vi "rszvl_core_global.vi"() -> ()   [LabVIEW 2014] (continued)
measured frequencies or whether an ENR list table is to be used (ENR values specified at specific input frequencies).\n\nAvailable Repeated Capabilities:\nNone\n\nRemote-control command(s):\n[SENSe]:CORRection:ENR:MODE[?] TABLe | SPOT", "Flags"={"OPC Wait"=FALSE, "Dont check status"=FALSE, "*WAI"=FALSE}, "Check Status Callback"=""}, {"Level"=3, "Descriptive Name"="Noise ERN Constant Value", "Class Only"=FALSE, "Data Type"=1, "Access"=2, "Identifier"="RSZVL_ATTR_NOISE_CORR_ENR_SPOT", "Range Table"="", "Command"="SENS:CORR:ENR:SPOT", "Read Callback"="", "Write Callback"="", "Range Callback"="", "Check Callback"="", "Rngtable Callback"="", "Coerce Callback"="", "User Callback"="", "Supported Models"="", "Instrument Options"="", "Repeated Capabilities"="", "Restricted Repeated Capabilities"="", "Help"="The ENR attribute allows the ENR value applicable to the Noise source for all input frequencies to be specified. This value provides a simple mechanism to enter an ENR value that is\napplicable throughout a range of measurement frequencies.\nThis attribute will however not be effective if\nthe remote control command SENS:CORR:ENR:MODE:TABL was previously entered.\n\nAvailable Repeated Capabilities:\nNone\n\nRemote-control command(s):\n[SENSe]:CORRection:ENR:SPOT[?] <numeric_value> [dB]", "Flags"={"OPC Wait"=FALSE, "Dont check status"=FALSE, "*WAI"=FALSE}, "Check Status Callback"=""}, {"Level"=3, "Descriptive Name"="Noise ENR Room Temperature", "Class Only"=FALSE, "Data Type"=1, "Access"=2, "Identifier"="RSZVL_ATTR_NOISE_CORR_TEMP", "Range Table"="", "Command"="SENS:CORR:TEMP", "Read Callback"="", "Write Callback"="", "Range Callback"="", "Check Callback"="", "Rngtable Callback"="", "Coerce Callback"="", "User Callback"="", "Supported Models"="", "Instrument Options"="", "Repeated Capabilities"="", "Restricted Repeated Capabilities"="", "Help"="This ENR attribute allows the room temperature of the operating environment to be specified. This value will be taken into account when calculating noise results. Units are Kelvin.\n\nAvailable Repeated Capabilities:\nNone\n\nRemote-control command(s):\n[SENSe]:CORRection:TEMPerature[?] <numeric_value> [K]", "Flags"={"OPC Wait"=FALSE, "Dont check status"=FALSE, "*WAI"=FALSE}, "Check Status Callback"=""}, {"Level"=3, "Descriptive Name"="Noise Loss Mode Selection", "Class Only"=FALSE, "Data Type"=0, "Access"=2, "Identifier"="RSZVL_ATTR_NOISE_CORR_LOSS_MODE", "Range Table"="rszvl_rngNoiseLossMode", "Command"="SENS:CORR:LOSS:{InputOutput}:MODE", "Read Callback"="", "Write Callback"="", "Range Callback"="", "Check Callback"="", "Rngtable Callback"="", "Coerce Callback"="", "User Callback"="", "Supported Models"="", "Instrument Options"="", "Repeated Capabilities"="", "Restricted Repeated Capabilities"="", "Help"="This attribute is used to identify whether a single input/output loss value applies for all measured frequencies or whether an input/output loss list is to be used. (Loss Input/Output values specified at specific input frequencies).\n\nAvailable Repeated Capabilities:\nInputOutput: Inp,Out\r\n\nRemote-control command(s):\n[SENSe]:CORRection:LOSS:INPut|OUTput:MODE[?] SPOT | TABLe", "Flags"={"OPC Wait"=FALSE, "Dont check status"=FALSE, "*WAI"=FALSE}, "Check Status Callback"=""}, {"Level"=3, "Descriptive Name"="Noise Loss Constant Value", "Class Only"=FALSE, "Data Type"=1, "Access"=2, "Identifier"="RSZVL_ATTR_NOISE_CORR_LOSS_SPOT", "Range Table"="", "Command"="SENS:CORR:LOSS:{InputOutput}:SPOT", "Read Callback"="", "Write Callback"="", "Range Callback"="", "Check Callback"="", "Rngtable Callback"="", "Coerce Callback"="", "User Callback"="", "Supported Models"="", "Instrument Options"="", "Repeated Capabilities"="", "Restricted Repeated Capabilities"="", "Help"="This attribute allows the loss input/output constant to be set to a value applicable for all input/output frequencies to be measured. This attribute provides a simple mechanism to enter a loss input/output value that is applicable throughout a range of measurement frequencies.\nThis attribute will however not be effective if the attribute RSZVL_ATTR_NOISE_CORR_LOSS_MODE - TABL was previously entered.\n\nAvailable Repeated Capabilities:\nInputOutput: Inp,Out\r\n\nRemote-control command(s):\n[SENSe]:CORRection:LOSS:<INPut|OUTPut>:SPOT[?] <numeric value> [dB]", "Flags"={"OPC Wait"=FALSE, "Dont check status"=FALSE, "*WAI"=FALSE}, "Check Status Callback"=""}, {"Level"=3, "Descriptive Name"="Noise Image Rejection", "Class Only"=FALSE, "Data Type"=1, "Access"=2, "Identifier"="RSZVL_ATTR_NOISE_CORR_EREJ", "Range Table"="", "Command"="SENS:CORR:IREJ", "Read Callback"="", "Write Callback"="", "Range Callback"="", "Check Callback"="", "Rngtable Callback"="", "Coerce Callback"="", "User Callback"="", "Supported Models"="", "Instrument Options"="", "Repeated Capabilities"="", "Restricted Repeated Capabilities"="", "Help"="This attribute allows an image rejection value associated with DUT to be entered which will be effective across the complete range of measurement frequencies.\n\nAvailable Repeated Capabilities:\nNone\n\nRemote-control command(s):\n[SENSe]:CORRection:IREJection[?] <numeric value > [dB]", "Flags"={"OPC Wait"=FALSE, "Dont check status"=FALSE, "*WAI"=FALSE}, "Check Status Callback"=""}, {"Level"=3, "Descriptive Name"="Noise 2nd State Correction", "Class Only"=FALSE, "Data Type"=3, "Access"=2, "Identifier"="RSZVL_ATTR_NOISE_CORR_STAT", "Range Table"="", "Command"="SENS:CORR:STAT", "Read Callback"="", "Write Callback"="", "Range Callback"="", "Check Callback"="", "Rngtable Callback"="", "Coerce Callback"="", "User Callback"="", "Supported Models"="", "Instrument Options"="", "Repeated Capabilities"="", "Restricted Repeated Capabilities"="", "Help"="This attribute can be used to control whether the R&S FS-K30 option will factor in the results obtained from second stage correction when performing a noise and gain measurement.\n\nAvailable Repeated Capabilities:\nNone\n\nRemote-control command(s):\n[SENSe]:CORRection[:STATe][?] ON | OFF", "Flags"={"OPC Wait"=FALSE, "Dont check status"=FALSE, "*WAI"=FALSE}, "Check Status Callback"=""}, {"Level"=3, "Descriptive Name"="Noise Frequency Step", "Class Only"=FALSE, "Data Type"=1, "Access"=2, "Identifier"="RSZVL_ATTR_NOISE_FREQ_STEP", "Range Table"="", "Command"="SENS:FREQ:STEP", "Read Callback"="", "Write Callback"="", "Range Callback"="", "Check Callback"="", "Rngtable Callback"="", "Coerce Callback"="", "User Callback"="", "Supported Models"="", "Instrument Options"="", "Repeated Capabilities"="", "Restricted Repeated Capabilities"="", "Help"="This attribute can be used to specify the step frequency for a new frequency measurement list that requires computing. This value will form the basis of one of the input criteria for computing a new frequency list.\n\nAvailable Repeated Capabilities:\nNone\n\nRemote-control command(s):\n[SENSe]:FREQuency:STEP[?] <numeric value> [Hz]", "Flags"={"OPC Wait"=FALSE, "Dont check status"=FALSE, "*WAI"=FALSE}, "Check Status Callback"=""}, {"Level"=3, "Descriptive Name"="Noise Fixed Frequency", "Class Only"=FALSE, "Data Type"=1, "Access"=2, "Identifier"="RSZVL_ATTR_NOISE_FREQ_FIXED", "Range Table"="", "Command"="SENS:FREQ:FIX", "Read Callback"="", "Write Callback"="", "Range Callback"="", "Check Callback"="", "Rngtable Callback"="", "Coerce Callback"="", "User Callback"="", "Supported Models"="", "Instrument Options"="", "Repeated Capabilities"="", "Restricted Repeated Capabilities"="", "Help"="This attribute is used to specify a single fixed frequency to measure noise and gain continuously. The value specified with this command is only used when a single frequency measurement is initiated.\n\nAvailable Repeated Capabilities:\nNone\n\nRemote-control command(s):\n[SENSe]:FREQuency[:CW|:FIXed][?] <numeric value> [Hz]", "Flags"={"OPC Wait"=FALSE, "Dont check status"=FALSE, "*WAI"=FALSE}, "Check Status Callback"=""}, {"Level"=3, "Descriptive Name"="Noise Fixed Local Oscilator Frequency", "Class Only"=FALSE, "Data Type"=1, "Access"=2, "Identifier"="RSZVL_ATTR_NOISE_CONF_SYST_LOSC_FREQ", "Range Table"="", "Command"="SENS:CONF:MODE:SYST:LOSC:FREQ", "Read Callback"="", "Write Callback"="", "Range Callback"="", "Check Callback"="", "Rngtable Callback"="", "Coerce Callback"="", "User Callback"="", "Supported Models"="", "Instrument Options"="", "Repeated Capabilities"="", "Restricted Repeated Capabilities"="", "Help"="This attribute can be used to specify a fixed local oscillator frequency for a new frequency measurement list that requires computing. This value will form the basis of one of the input criteria for computing a new frequency list.\nThe attribute will not have any immediate effect if a direct frequency list is being used (which is set by the RSZVL_ATTR_NOISE_CONF_MODE_DUT - AMPL attribute) or a variable local osciallator frequency has been specified (which is set by the RSZVL_ATTR_NOISE_CONF_SYST_LOSC - VAR attribute).\n\nAvailable Repeated Capabilities:\nNone\n\nRemote-control command(s):\n[SENSe]:CONFigure:MODE:SYSTem:LOSCillator:FREQuency[?] <numeric value> [Hz]", "Flags"={"OPC Wait"=FALSE, "Dont check status"=FALSE, "*WAI"=FALSE}, "Check Status Callback"=""}, {"Level"=3, "Descriptive Name"="Noise Configure DUT", "Class Only"=FALSE, "Data Type"=0, "Access"=2, "Identifier"="RSZVL_ATTR_NOISE_CONF_MODE_DUT", "Range Table"="rszvl_rngNoiseConfDUT", "Command"="SENS:CONF:MODE:DUT", "Read Callback"="", "Write Callback"="", "Range Callback"="", "Check Callback"="", "Rngtable Callback"="", "Coerce Callback"="", "User Callback"="", "Supported Models"="", "Instrument Options"="", "Repeated Capabilities"="", "Restricted Repeated Capabilities"="", "Help"="This attribute allows the type of DUT to be defined. This setting will determine the method that will be used to create the frequency measurement list. This attribute in addition to Noise Configure Local Oscilator will determine how the DUT is tested. Fixed Local Oscillator or fixed Intermediate Frequencies will be taken from the settings supplied by its functions, where appropriate.\nThe following calculation methods will be used.\nUsing a variable Local Oscillator frequency as set by the attribute RSZVL_ATTR_NOISE_CONF_SYST_LOSC - VAR: i.e. the DUT has a fixed IF frequency.\nUsing a fixed Local Oscillator frequency as set by the attribute RSZVL_ATTR_NOISE_CONF_SYST_LOSC -\nFIX: i.e. the DUT has a variable IF frequency.\nThe attribute will not have any immediate effect if the current frequency measurement mode is\nfixed, as is set by the command SENS:FREQ:MODE FIX.\nRF: = All the above settings for frequency list calculation will calculate the RF frequency for each step.\nThe list of RF frequencies generated will be in the following sequence: Start Frequency, Start\nFrequency + Step Frequency, Start Frequency + Step Frequency*2, Stop Frequency.\nIF: = intermediate frequency\nLO: = local oscillator frequency\n\nAvailable Repeated Capabilities:\nNone\n\nRemote-control command(s):\n[SENSe]:CONFigure:MODE:DUT[?] AMPLifier | DOWNc | UPConv", "Flags"={"OPC Wait"=FALSE, "Dont check status"=FALSE, "*WAI"=FALSE}, "Check Status Callback"=""}, {"Level"=3, "Descriptive Name"="Noise Configure Range", "Class Only"=FALSE, "Data Type"=1, "Access"=2, "Identifier"="RSZVL_ATTR_NOISE_CONF_DUT_GAIN", "Range Table"="", "Command"="SYST:CONF:DUT:GAIN", "Read Callback"="", "Write Callback"="", "Range Callback"="", "Check Callback"="", "Rngtable Callback"="", "Coerce Callback"="", "User Callback"="", "Supported Models"="", "Instrument Options"="", "Repeated Capabilities"="", "Restricted Repeated Capabilities"="", "Help"="This attribute allows the maximum gain of the DUT to be specified.\n\nAvailable Repeated Capabilities:\nNone\n\nRemote-control command(s):\nSYSTem:CONFigure:DUT:GAIN[?] <numeric value> [dB]", "Flags"={"OPC Wait"=FALSE, "Dont check status"=FALSE, "*WAI"=FALSE}, "Check Status Callback"=""}, {"Level"=3, "Descriptive Name"="Noise Settling Time", "Class Only"=FALSE, "Data Type"=1, "Access"=2, "Identifier"="RSZVL_ATTR_NOISE_CONF_DUT_SETT_TIME", "Range Table"="", "Command"="SYST:CONF:DUT:STIM", "Read Callback"="", "Write Callback"="", "Range Callback"="", "Check Callback"="", "Rngtable Callback"="", "Coerce Callback"="", "User Callback"="", "Supported Models"="", "Instrument Options"="", "Repeated Capabilities"="", "Restricted Repeated Capabilities"="", "Help"="This attribute allows the DUT settling time to be modified. It represents the time to wait for the DUT to settle after a noise source has been turned on or off.\n\nAvailable Repeated Capabilities:\nNone\n\nRemote-control command(s):\nSYSTem:CONFigure:DUT:STIMe[?] <numeric value> [s]", "Flags"={"OPC Wait"=FALSE, "Dont check status"=FALSE, "*WAI"=FALSE}, "Check Status Callback"=""}, {"Level"=3, "Descriptive Name"="Noise Save Trace To Memory", "Class Only"=FALSE, "Data Type"=4, "Access"=1, "Identifier"="RSZVL_ATTR_NOISE_ARRAY_MEMORY", "Range Table"="", "Command"="CONF:ARR:MEM{NoiseTraceMemory} ONCE", "Read Callback"="", "Write Callback"="", "Range Callback"="", "Check Callback"="", "Rngtable Callback"="", "Coerce Callback"="", "User Callback"="", "Supported Models"="", "Instrument Options"="", "Repeated Capabilities"="", "Restricted Repeated Capabilities"="", "Help"="This attribute saves the current trace results (noise figure, noise temperature and noise gain traces) to trace memory <n>.\n\nAvailable Repeated Capabilities:\nNoiseTraceMemory: MEM1,MEM2,MEM3\r\n\nRemote-control command(s):\nCONFigure:ARRay:MEMory<1...3> ONCE", "Flags"={"OPC Wait"=FALSE, "Dont check status"=FALSE, "*WAI"=FALSE}, "Check Status Callback"=""}, {"Level"=3, "Descriptive Name"="Noise Assign Marker To Trace", "Class Only"=FALSE, "Data Type"=0, "Access"=2, "Identifier"="RSZVL_ATTR_NOISE_MARKER_TRACE", "Range Table"="rszvl_rngNoiseMarkerTrace", "Command"="CALC:MARK:TRAC", "Read Callback"="", "Write Callback"="", "Range Callback"="", "Check Callback"="", "Rngtable Callback"="", "Coerce Callback"="", "User Callback"="", "Supported Models"="", "Instrument Options"="", "Repeated Capabilities"="", "Restricted Repeated Capabilities"="", "Help"="This attribute assigns the marker1 to the indicated trace.\n\nAvailable Repeated Capabilities:\nNone\n\nRemote-control command(s):\nCALCulate:MARKer:TRACe NOISe | GAIN", "Flags"={"OPC Wait"=FALSE, "Dont check status"=FALSE, "*WAI"=FALSE}, "Check Status Callback"=""}, {"Level"=2, "Descriptive Name"="Display", "Class Only"=TRUE, "Data Type"=0, "Access"=0, "Identifier"="", "Range Table"="", "Command"="", "Read Callback"="", "Write Callback"="", "Range Callback"="", "Check Callback"="", "Rngtable Callback"="", "Coerce Callback"="", "User Callback"="", "Supported Models"="", "Instrument Options"="", "Repeated Capabilities"="", "Restricted Repeated Capabilities"="", "Help"="Attributes that configure the display parameters.\n\n(1) Noise Display Y-Axis Trace Type:\nThis attribute allows the user to specify the type of data to be displayed in trace 1. The user can select either to display either Noise Figure results (NFIGure) or Noise temperature (TEFFective – to keep compatibility with the NFA). Note that Trace 1 is always noise results and Trace 2 is always for Gain results.\n\n(2) Noise Display Trace State:\nThis attribute switches on or off the display of the corresponding trace and related information in\nthe selected measurement window.\n\n(3) Noise Display Symbols:\nThis attribute switches on or off the display of the symbols to mark the measurement points for the\nspecified trace i.e. Noise or Gain.\nThis attribute will only have a noticeable effect if the required trace is active as set by the\nattribute RSZVL_ATTR_NOISE_DISP_TRAC_STAT ON.\n\n(4) Noise Automatic Scaling:\nThis attribute switches on or off automatic scaling of the Y-axis for the specified trace display.\nAutomatic scaling set the Y-axis to automatically scale to best fit the measurement results.\nNote that the specified trace must be active for this attribute to have an immediate effect. This can be achieved using the attribute RSZVL_ATTR_NOISE_DISP_TRAC_STAT ON.\n\n(5) Noise Minimum Y-Axis Value:\nThis attribute sets the minimum (bottom) Y-axis display value for the specified trace display. Note that this attribute has no affect if automatic scaling of the Y-axis is enabled or the specified trace is not currently active.\n\n(6) Noise Maximum Y-Axis Value:\nThis attribute sets the maximum (top) Y-axis display value for the specified trace display. Note that this attribute has no affect if automatic scaling of the Y-axis is enabled or the specified trace is not currently active.\n\n(7) Noise Automatic Reference Level:\nThis attribute enables or disables automatic reference level detection.\n\n(8) Noise Display Table:\nThis attribute toggles the display of results in graphical or tabular form.\n\n(9) Noise Display Trace Memory:\nswitches the display of trace memory <n> on or off.\nThis command is available from firmware version 1.60.\n\n(10) Noise Display Current Results State:\nThis attribute switches the display of the current measurement results on or off.\nThis command is available from firmware version 1.60.\n\n(11) Noise X-Axis Frequency Display:\nThis attribute selects the frequency to be displayed on the x–axis if the DUT is not an amplifier, i.e. in a frequency–converting measurement mode.", "Flags"={"OPC Wait"=FALSE, "Dont check status"=FALSE, "*WAI"=FALSE}, "Check Status Callback"=""}, {"Level"=3, "Descriptive Name"="Noise Display Y-Axis Trace Type", "Class Only"=FALSE, "Data Type"=0, "Access"=2, "Identifier"="RSZVL_ATTR_NOISE_DISP_DATA_TRAC", "Range Table"="rszvl_rngNoiseDispDataTrac", "Command"="DISP:DATA:TRAC{Trace}", "Read Callback"="", "Write Callback"="", "Range Callback"="", "Check Callback"="", "Rngtable Callback"="", "Coerce Callback"="", "User Callback"="", "Supported Models"="", "Instrument Options"="", "Repeated Capabilities"="", "Restricted Repeated Capabilities"="", "Help"="This attribute allows the user to specify the type of data to be displayed in trace 1. The user can select either to display either Noise Figure results (NFIGure) or Noise temperature (TEFFective – to keep compatibility with the NFA). Note that Trace 1 is always noise results and Trace 2 is always for Gain results.\n\nAvailable Repeated Capabilities:\nTrace: TR1,TR2,TR3,TR4,TR5,TR6,TR7,TR8,TR9,TR10,TR11,TR12,TR13,TR14,TR15,TR16,TR17,TR18,TR19,TR20\r\n\nRemote-control command(s):\nDISPlay:DATA:TRACe<1>[?] NFIGure | TEFFective", "Flags"={"OPC Wait"=FALSE, "Dont check status"=FALSE, "*WAI"=FALSE}, "Check Status Callback"=""}, {"Level"=3, "Descriptive Name"="Noise Display Trace State", "Class Only"=FALSE, "Data Type"=3, "Access"=2, "Identifier"="RSZVL_ATTR_NOISE_DISP_TRAC_STAT", "Range Table"="", "Command"="DISP:TRAC{Trace}", "Read Callback"="", "Write Callback"="", "Range Callback"="", "Check Callback"="", "Rngtable Callback"="", "Coerce Callback"="", "User Callback"="", "Supported Models"="", "Instrument Options"="", "Repeated Capabilities"="", "Restricted Repeated Capabilities"="", "Help"="This attribute switches on or off the display of the corresponding trace and related information in\nthe selected measurement window.\n\nAvailable Repeated Capabilities:\nTrace: TR1,TR2,TR3,TR4,TR5,TR6,TR7,TR8,TR9,TR10,TR11,TR12,TR13,TR14,TR15,TR16,TR17,TR18,TR19,TR20\r\n\nRemote-control command(s):\nDISPlay[:WINDow<1>]:TRACe<1|2>[:STATe][?] ON | OFF", "Flags"={"OPC Wait"=FALSE, "Dont check status"=FALSE, "*WAI"=FALSE}, "Check Status Callback"=""}, {"Level"=3, "Descriptive Name"="Noise Display Symbols", "Class Only"=FALSE, "Data Type"=3, "Access"=2, "Identifier"="RSZVL_ATTR_NOISE_DISP_SYMB", "Range Table"="", "Command"="DISP:TRAC{Trace}:SYMB", "Read Callback"="", "Write Callback"="", "Range Callback"="", "Check Callback"="", "Rngtable Callback"="", "Coerce Callback"="", "User Callback"="", "Supported Models"="", "Instrument Options"="", "Repeated Capabilities"="", "Restricted Repeated Capabilities"="", "Help"="This attribute switches on or off the display of the symbols to mark the measurement points for the\nspecified trace i.e. Noise or Gain.\nThis attribute will only have a noticeable effect if the required trace is active as set by the\nattribute RSZVL_ATTR_NOISE_DISP_TRAC_STAT ON.\n\nAvailable Repeated Capabilities:\nTrace: TR1,TR2,TR3,TR4,TR5,TR6,TR7,TR8,TR9,TR10,TR11,TR12,TR13,TR14,TR15,TR16,TR17,TR18,TR19,TR20\r\n\nRemote-control command(s):\nDISPlay[:WINDow<1>]:TRACe<1|2>:SYMBols[?] ON | OFF", "Flags"={"OPC Wait"=FALSE, "Dont check status"=FALSE, "*WAI"=FALSE}, "Check Status Callback"=""}, {"Level"=3, "Descriptive Name"="Noise Automatic Scaling", "Class Only"=FALSE, "Data Type"=3, "Access"=2, "Identifier"="RSZVL_ATTR_NOISE_DISP_AUTO_SCAL", "Range Table"="", "Command"="DISP:TRAC{Trace}:Y:AUTO", "Read Callback"="", "Write Callback"="", "Range Callback"="", "Check Callback"="", "Rngtable Callback"="", "Coerce Callback"="", "User Callback"="", "Supported Models"="", "Instrument Options"="", "Repeated Capabilities"="", "Restricted Repeated Capabilities"="", "Help"="This attribute switches on or off automatic scaling of the Y-axis for the specified trace display.\nAutomatic scaling set the Y-axis to automatically scale to best fit the measurement results.\nNote that the specified trace must be active for this attribute to have an immediate effect. This can be achieved using the attribute RSZVL_ATTR_NOISE_DISP_TRAC_STAT ON.\n\nAvailable Repeated Capabilities:\nTrace: TR1,TR2,TR3,TR4,TR5,TR6,TR7,TR8,TR9,TR10,TR11,TR12,TR13,TR14,TR15,TR16,TR17,TR18,TR19,TR20\r\n\nRemote-control command(s):\nDISPlay[:WINDow<1>]:TRACe<1|2>:Y[:SCALe]:AUTO[?] ON | OFF", "Flags"={"OPC Wait"=FALSE, "Dont check status"=FALSE, "*WAI"=FALSE}, "Check Status Callback"=""}, {"Level"=3, "Descriptive Name"="Noise Minimum Y-Axis Value", "Class Only"=FALSE, "Data Type"=1, "Access"=2, "Identifier"="RSZVL_ATTR_NOISE_DISP_TRAC_BOTTOM", "Range Table"="", "Command"="DISP:TRAC{Trace}:Y:BOTT", "Read Callback"="", "Write Callback"="", "Range Callback"="", "Check Callback"="", "Rngtable Callback"="", "Coerce Callback"="", "User Callback"="", "Supported Models"="", "Instrument Options"="", "Repeated Capabilities"="", "Restricted Repeated Capabilities"="", "Help"="This attribute sets the minimum (bottom) Y-axis display value for the specified trace display. Note that this attribute has no affect if automatic scaling of the Y-axis is enabled or the specified trace is not currently active.\n\nAvailable Repeated Capabilities:\nTrace: TR1,TR2,TR3,TR4,TR5,TR6,TR7,TR8,TR9,TR10,TR11,TR12,TR13,TR14,TR15,TR16,TR17,TR18,TR19,TR20\r\n\nRemote-control command(s):\nDISPlay[:WINDow<1>]:TRACe<1|2>:Y[:SCALe]:BOTTom[?] <numeric_value> [dB]", "Flags"={"OPC Wait"=FALSE, "Dont check status"=FALSE, "*WAI"=FALSE}, "Check Status Callback"=""}, {"Level"=3, "Descriptive Name"="Noise Maximum Y-Axis Value", "Class Only"=FALSE, "Data Type"=1, "Access"=2, "Identifier"="RSZVL_ATTR_NOISE_DISP_TRAC_TOP", "Range Table"="", "Command"="DISP:TRAC{Trace}:Y:TOP", "Read Callback"="", "Write Callback"="", "Range Callback"="", "Check Callback"="", "Rngtable Callback"="", "Coerce Callback"="", "User Callback"="", "Supported Models"="", "Instrument Options"="", "Repeated Capabilities"="", "Restricted Repeated Capabilities"="", "Help"="This attribute sets the maximum (top) Y-axis display value for the specified trace display. Note that this attribute has no affect if automatic scaling of the Y-axis is enabled or the specified trace is not currently active.\n\nAvailable Repeated Capabilities:\nTrace: TR1,TR2,TR3,TR4,TR5,TR6,TR7,TR8,TR9,TR10,TR11,TR12,TR13,TR14,TR15,TR16,TR17,TR18,TR19,TR20\r\n\nRemote-control command(s):\nDISPlay[:WINDow<1>]:TRACe<1|2>:Y[:SCALe]:TOP[?] <numeric_value> [dB]", "Flags"={"OPC Wait"=FALSE, "Dont check status"=FALSE, "*WAI"=FALSE}, "Check Status Callback"=""}, {"Level"=3, "Descriptive Name"="Noise Automatic Reference Level", "Class Only"=FALSE, "Data Type"=3, "Access"=2, "Identifier"="RSZVL_ATTR_NOISE_DISP_TRAC_REF_LEV_STAT", "Range Table"="", "Command"="DISP:TRAC{Trace}:Y:RLEV:AUTO", "Read Callback"="", "Write Callback"="", "Range Callback"="", "Check Callback"="", "Rngtable Callback"="", "Coerce Callback"="", "User Callback"="", "Supported Models"="", "Instrument Options"="", "Repeated Capabilities"="", "Restricted Repeated Capabilities"="", "Help"="This attribute enables or disables automatic reference level detection.\n\nAvailable Repeated Capabilities:\nTrace: TR1,TR2,TR3,TR4,TR5,TR6,TR7,TR8,TR9,TR10,TR11,TR12,TR13,TR14,TR15,TR16,TR17,TR18,TR19,TR20\r\n\nRemote-control command(s):\nDISPlay[:WINDow<1>]:TRACe<1|2>:Y[:SCALe]:RLEVel:AUTO[?] ON | OFF", "Flags"={"OPC Wait"=TRUE, "Dont check status"=FALSE, "*WAI"=FALSE}, "Check Status Callback"=""}, {"Level"=3, "Descriptive Name"="Display Format", "Class Only"=FALSE, "Data Type"=0, "Access"=2, "Identifier"="RSZVL_ATTR_NOISE_DISP_FORMAT", "Range Table"="rszvl_rngDISPFormat", "Command"="DISP:FORM", "Read Callback"="", "Write Callback"="", "Range Callback"="", "Check Callback"="", "Rngtable Callback"="", "Coerce Callback"="", "User Callback"="", "Supported Models"="", "Instrument Options"="", "Repeated Capabilities"="", "Restricted Repeated Capabilities"="", "Help"="This attribute switches the measurement result display between FULL SCREEN and SPLIT SCREEN. The coupling of settings between screen A and screen B can be selected with the command INSTrument:COUPle.\n\nAvailable Repeated Capabilities:\nNone\n\nRemote-control command(s):\nDISPlay:FORMat SINGle | SPLit", "Flags"={"OPC Wait"=FALSE, "Dont check status"=FALSE, "*WAI"=FALSE}, "Check Status Callback"=""}, {"Level"=3, "Descriptive Name"="Noise Display Table", "Class Only"=FALSE, "Data Type"=3, "Access"=2, "Identifier"="RSZVL_ATTR_NOISE_DISP_TABLE", "Range Table"="", "Command"="DISP:TABL", "Read Callback"="", "Write Callback"="", "Range Callback"="", "Check Callback"="", "Rngtable Callback"="", "Coerce Callback"="", "User Callback"="", "Supported Models"="", "Instrument Options"="", "Repeated Capabilities"="", "Restricted Repeated Capabilities"="", "Help"="This attribute toggles the display of results in graphical or tabular form.\n\nAvailable Repeated Capabilities:\nNone\n\nRemote-control command(s):\nDISPlay[:WINDow<1>]:TABLe[?] ON | OFF", "Flags"={"OPC Wait"=FALSE, "Dont check status"=FALSE, "*WAI"=FALSE}, "Check Status Callback"=""}, {"Level"=3, "Descriptive Name"="Noise Display Trace Memory", "Class Only"=FALSE, "Data Type"=3, "Access"=2, "Identifier"="RSZVL_ATTR_NOISE_DISP_TRACE_MEM", "Range Table"="", "Command"="DISP:ARR:MEM{NoiseTraceMemory}", "Read Callback"="", "Write Callback"="", "Range Callback"="", "Check Callback"="", "Rngtable Callback"="", "Coerce Callback"="", "User Callback"="", "Supported Models"="", "Instrument Options"="", "Repeated Capabilities"="", "Restricted Repeated Capabilities"="", "Help"="switches the display of trace memory <n> on or off.\nThis command is available from firmware version 1.60.\n\nAvailable Repeated Capabilities:\nNoiseTraceMemory: MEM1,MEM2,MEM3\r\n\nRemote-control command(s):\nDISPlay:ARRay:MEMory<1...3>[:STATe]", "Flags"={"OPC Wait"=FALSE, "Dont check status"=FALSE, "*WAI"=FALSE}, "Check Status Callback"=""}, {"Level"=3, "Descriptive Name"="Noise Display Current Results State", "Class Only"=FALSE, "Data Type"=3, "Access"=2, "Identifier"="RSZVL_ATTR_NOISE_DISPL_CURR_RESULTS", "Range Table"="", "Command"="DISP:CURR:DATA", "Read Callback"="", "Write Callback"="", "Range Callback"="", "Check Callback"="", "Rngtable Callback"="", "Coerce Callback"="", "User Callback"="", "Supported Models"="", "Instrument Options"="", "Repeated Capabilities"="", "Restricted Repeated Capabilities"="", "Help"="This attribute switches the display of the current measurement results on or off.\nThis command is available from firmware version 1.60.\n\nAvailable Repeated Capabilities:\nNone\n\nRemote-control command(s):\nDISPlay:CURRent:DATA[:STATe] OFF | ON", "Flags"={"OPC Wait"=FALSE, "Dont check status"=FALSE, "*WAI"=FALSE}, "Check Status Callback"=""}, {"Level"=3, "Descriptive Name"="Noise X-Axis Frequency Display", "Class Only"=FALSE, "Data Type"=0, "Access"=2, "Identifier"="RSZVL_ATTR_NOISE_DISP_X_AXIS", "Range Table"="rszvl_rngNoiseXAxisFrequency", "Command"="DISP:TRAC{Trace}:X", "Read Callback"="", "Write Callback"="", "Range Callback"="", "Check Callback"="", "Rngtable Callback"="", "Coerce Callback"="", "User Callback"="", "Supported Models"="", "Instrument Options"="", "Repeated Capabilities"="", "Restricted Repeated Capabilities"="", "Help"="This attribute selects the frequency to be displayed on the x–axis if the DUT is not an amplifier, i.e. in a frequency–converting measurement mode.\n\nAvailable Repeated Capabilities:\nTrace: TR1,TR2,TR3,TR4,TR5,TR6,TR7,TR8,TR9,TR10,TR11,TR12,TR13,TR14,TR15,TR16,TR17,TR18,TR19,TR20\r\n\nRemote-control command(s):\nDISPlay[:WINDow<1>]:TRACe<1|2>:X[:SCALe]", "Flags"={"OPC Wait"=FALSE, "Dont check status"=FALSE, "*WAI"=FALSE}, "Check Status Callback"=""}, {"Level"=1, "Descriptive Name"="K72 - 3GPP FDD Base Station Test", "Class Only"=TRUE, "Data Type"=0, "Access"=0, "Identifier"="", "Range Table"="", "Command"="", "Read Callback"="", "Write Callback"="", "Range Callback"="", "Check Callback"="", "Rngtable Callback"="", "Coerce Callback"="", "User Callback"="", "Supported Models"="", "Instrument Options"="", "Repeated Capabilities"="", "Restricted Repeated Capabilities"="", "Help"="This class implements attributes of options K72 - 3GPP FDD Base Station Test.\n\n(1) 3GPP BS Mode:\nThis attribute sets the instrument to the 3GPP BS Mode.\n\n(2) 3GPP BS FSL Mode (BWCD):\nThis attribute sets the instrument to the 3GPP BS (BWCD) Mode.\n\n(3) 3GPP BS Measurement:\nThis attribute selects the 3GPP FDD base station tests.\n\n(4) WCDP (Class):\nAttributes that configure the WCDP measurement.\n\n(5) MCACLR (Class):\nAttributes that configure the multicarrier ACLR measurement.\n\n\n(6) Settings (Class):\nAttributes that configure the common settings.\n\n(7) Channel Table Configuration (Class):\nAttributes that configure the channel table.\n\n(8) Results (Class):\nAttributes that returns the measurement results.", "Flags"={"OPC Wait"=FALSE, "Dont check status"=FALSE, "*WAI"=FALSE}, "Check Status Callback"=""}, {"Level"=2, "Descriptive Name"="3GPP BS Mode", "Class Only"=FALSE, "Data Type"=4, "Access"=1, "Identifier"="RSZVL_ATTR_BWCD_MODE", "Range Table"="", "Command"="INST BWCD", "Read Callback"="", "Write Callback"="", "Range Callback"="", "Check Callback"="", "Rngtable Callback"="", "Coerce Callback"="", "User Callback"="", "Supported Models"="", "Instrument Options"="", "Repeated Capabilities"="", "Restricted Repeated Capabilities"="", "Help"="This attribute sets the instrument to the 3GPP BS (BWCD) Mode.\n\nAvailable Repeated Capabilities:\nNone\n\nRemote-control command(s):\nINSTrument[:SELect] BWCD", "Flags"={"OPC Wait"=FALSE, "Dont check status"=FALSE, "*WAI"=FALSE}, "Check Status Callback"=""}, {"Level"=2, "Descriptive Name"="3GPP BS Measurement", "Class Only"=FALSE, "Data Type"=0, "Access"=2, "Identifier"="RSZVL_ATTR_3GBS_MEAS", "Range Table"="rszvl_rng3GBSMeas", "Command"="CONF:WCDP:MEAS", "Read Callback"="", "Write Callback"="", "Range Callback"="", "Check Callback"="", "Rngtable Callback"="", "Coerce Callback"="", "User Callback"="", "Supported Models"="", "Instrument Options"="", "Repeated Capabilities"="", "Restricted Repeated Capabilities"="", "Help"="This attribute selects the 3GPP FDD base station tests.\n\nAvailable Repeated Capabilities:\nNone\n\nRemote-control command(s):\nCONFigure<1>:WCDPower[:BTS]:MEASurement POWer | ACLR | ESPectrum | WCDPower", "Flags"={"OPC Wait"=FALSE, "Dont check status"=FALSE, "*WAI"=FALSE}, "Check Status Callback"=""}, {"Level"=2, "Descriptive Name"="3GPP BS Adjust Reference Level", "Class Only"=FALSE, "Data Type"=4, "Access"=1, "Identifier"="RSZVL_ATTR_3GPP_LEVEL_ADJUST", "Range Table"="", "Command"="SENS:CDP:LEV:ADJ", "Read Callback"="", "Write Callback"="", "Range Callback"="", "Check Callback"="", "Rngtable Callback"="", "Coerce Callback"="", "User Callback"="", "Supported Models"="", "Instrument Options"="", "Repeated Capabilities"="", "Restricted Repeated Capabilities"="", "Help"="This attribute adjusts the reference level to the measured channel power. This ensures that the settings of the RF attenuation and the reference level are optimally adjusted to the signal level without overloading the R&S ZVL or limiting the dynamic range by an S/N ratio that is too small.\n\nAvailable Repeated Capabilities:\nNone\n\nRemote-control command(s):\n[SENSe<1|2>:]CDPower:LEVel:ADJust", "Flags"={"OPC Wait"=TRUE, "Dont check status"=FALSE, "*WAI"=FALSE}, "Check Status Callback"=""}, {"Level"=2, "Descriptive Name"="WCDP", "Class Only"=TRUE, "Data Type"=0, "Access"=0, "Identifier"="", "Range Table"="", "Command"="", "Read Callback"="", "Write Callback"="", "Range Callback"="", "Check Callback"="", "Rngtable Callback"="", "Coerce Callback"="", "User Callback"="", "Supported Models"="", "Instrument Options"="", "Repeated Capabilities"="", "Restricted Repeated Capabilities"="", "Help"="Attributes that configure the WCDP measurement.\n\n(1) 3GPP BS Measurement WCDP HS-DPA/UPA State:\nThis attribute selects if the HS-DPCCH channel is searched or not.\n\nON: The high speed channels can be detected.\nA detection of the modulation typ (QPSK /16QAM) is done instead of a detection of pilot\nsymbols.\nOFF: The high speed channel can not be detected.\nA detection of pilot symbols is done instead a detection of the modulation typ (QPSK\n/16QAM).\n\n(2) 3GPP BS Measurement WCDP Settings Synchronization Type:\nThis attribute selects the type of synchronization.\nCPICH Synchronization to CPICH (default setting). For this type of synchronization, the CPICH\nmust be present in the transmit signal.\nSCH Synchronization without CPICH. This type of synchronization is required for test model 4\nwithout CPICH.\n\n(3) 3GPP BS Measurement WCDP Settings Auto Scale:\nThis attribute sets the autoscale state . It is available if multi carrier is switched ON. \n\nON Changes the level settings, if the center frequency is changed to another carrier.\n\nOFF Does not change the level settings, if the center frequency is changed to another carrier.\n\n(4) 3GPP BS Measurement WCDP Settings Multi Carrier:\nIf multi carrier is switched ON, the adjust reference level procedure ensures that the settings of RF attenuation and reference level are optimally adjusted for measuring a multi carrier signal.\n\nON Adjust reference level considering multi carrier conditions.\nOFF Adjust reference level considering single carrier conditions\n\n(5) 3GPP BS Measurement WCDP Settings Normalize:\nThis attribute switches elimination of I/Q offset on or off.\n\n(6) 3GPP BS Measurement WCDP Settings Compare Mode:\nThis attribute determines the power control measurement position. The slot power can be\naveraged from the beginning of the slot to the end of the slot (param. SLOT) or from the beginning of\nthe pilot symbols of the previous slot to the beginning of the pilot symbols of the actual slot. (param. PILOT). Furthermore, an enhanced channel search is used to consider the properties of\ncompressed mode channels.\n\n(7) 3GPP BS Measurement WCDP Settings Invert Q:\nThis attribute inverts the Q component of the signal.\n\n(8) 3GPP BS Measurement WCDP Settings Power Reference:\nThis attribute switches between the use of total power or CPICH power as the reference for the\nrelative CDP measurement values.\n\n(9) 3GPP BS Measurement WCDP Settings Side Band:\nThis attribute is for interchanging the left and the right sidebands.\n\n(10) 3GPP BS Measurement WCDP Settings Inactive Channel Treshold:\nThis attribute sets the threshold value from which a channel is treated as active. The level entered\nrefers to the total signal power.\n\n(11) 3GPP BS Measurement WCDP Power Difference:\nThis attribute activates or deactivates the slot power difference calculation of the POWER VERSUS SLOT display.\n\nON The slot power difference to the previous slot is displayed (POWER VS SLOT display).\nOFF The slot power of each slot is displayed (POWER VS SLOT display).\n\n(12) 3GPP BS Measurement WCDP Constellation Parameter B:\nThis attribute selects the constellation parameter B. According to 3GPP specification the mapping\nof 16QAM symbols to an assigned bit pattern depends on the constellation parameter B.\n\n(13) 3GPP BS Measurement WCDP Multiframe Capture Length:\nThis attribute specifies the number of frames that are captured by one sweep.\n\nRange: R&S FSU / R&S FSP-B70 (free run): [1 ... 2]\nR&S FSU / R&S FSP-B70 (ext. trig): [1 ... 3]\nR&S FSQ: [1 ... 100]\n\n(14) 3GPP BS Measurement WCDP Multiframe Frame To Analyze:\nThis attribute sets the frame number to be analyzed.", "Flags"={"OPC Wait"=FALSE, "Dont check status"=FALSE, "*WAI"=FALSE}, "Check Status Callback"=""}, {"Level"=3, "Descriptive Name"="3GPP BS Measurement WCDP HS-DPA/UPA State", "Class Only"=FALSE, "Data Type"=3, "Access"=2, "Identifier"="RSZVL_ATTR_3GBS_WCDP_HSDPAUPA_STATE", "Range Table"="", "Command"="CDP:HSDP", "Read Callback"="", "Write Callback"="", "Range Callback"="", "Check Callback"="", "Rngtable Callback"="", "Coerce Callback"="", "User Callback"="", "Supported Models"="", "Instrument Options"="", "Repeated Capabilities"="", "Restricted Repeated Capabilities"="", "Help"="This attribute selects if the HS-DPCCH channel is searched or not.\n\nON: The high speed channels can be detected.\nA detection of the modulation typ (QPSK /16QAM) is done instead of a detection of pilot\nsymbols.\nOFF: The high speed channel can not be detected.\nA detection of pilot symbols is done instead a detection of the modulation typ (QPSK\n/16QAM).\n\nAvailable Repeated Capabilities:\nNone\n\nRemote-control command(s):\n[SENSe:]CDPower:HSDPamode ON|OFF", "Flags"={"OPC Wait"=FALSE, "Dont check status"=FALSE, "*WAI"=FALSE}, "Check Status Callback"=""}, {"Level"=3, "Descriptive Name"="3GPP BS Measurement WCDP Settings Synchronization Type", "Class Only"=FALSE, "Data Type"=0, "Access"=2, "Identifier"="RSZVL_ATTR_3GBS_WCDP_SYNC_TYPE", "Range Table"="rszvl_rng3GBSSyncType", "Command"="CDP:STYPE", "Read Callback"="", "Write Callback"="", "Range Callback"="", "Check Callback"="", "Rngtable Callback"="", "Coerce Callback"="", "User Callback"="", "Supported Models"="", "Instrument Options"="", "Repeated Capabilities"="", "Restricted Repeated Capabilities"="", "Help"="This attribute selects the type of synchronization.\nCPICH Synchronization to CPICH (default setting). For this type of synchronization, the CPICH\nmust be present in the transmit signal.\nSCH Synchronization without CPICH. This type of synchronization is required for test model 4\nwithout CPICH.\n\nAvailable Repeated Capabilities:\nNone\n\nRemote-control command(s):\n[SENSe<1|2>:]CDPower:STYPe CPICh | SCHannel", "Flags"={"OPC Wait"=FALSE, "Dont check status"=FALSE, "*WAI"=FALSE}, "Check Status Callback"=""}, {"Level"=3, "Descriptive Name"="3GPP BS Measurement WCDP Settings Normalize", "Class Only"=FALSE, "Data Type"=3, "Access"=2, "Identifier"="RSZVL_ATTR_3GBS_WCDP_NORMALIZE", "Range Table"="", "Command"="CDP:NORM", "Read Callback"="", "Write Callback"="", "Range Callback"="", "Check Callback"="", "Rngtable Callback"="", "Coerce Callback"="", "User Callback"="", "Supported Models"="", "Instrument Options"="", "Repeated Capabilities"="", "Restricted Repeated Capabilities"="", "Help"="This attribute switches elimination of I/Q offset on or off.\n\nAvailable Repeated Capabilities:\nNone\n\nRemote-control command(s):\n[SENSe:]CDPower:NORMalize ON | OFF", "Flags"={"OPC Wait"=FALSE, "Dont check status"=FALSE, "*WAI"=FALSE}, "Check Status Callback"=""}, {"Level"=3, "Descriptive Name"="3GPP BS Measurement WCDP Settings Invert Q", "Class Only"=FALSE, "Data Type"=3, "Access"=2, "Identifier"="RSZVL_ATTR_3GBS_WCDP_INVERT_Q", "Range Table"="", "Command"="CDP:QINV", "Read Callback"="", 
